vi "打开数据库.vi"(8 "error in (no error)":errorcluster, 11 "sqlerver in":refnum<class "sqlerver.lvclass">) -> (0 "error out":errorcluster, 3 "sqlerver out":refnum<class "sqlerver.lvclass">)   [LabVIEW 2016, in "sqlerver.lvclass"]
uses:
  sqlerver.lvclass
  sqlerver.lvclass/sqlerver.ctl
  <vilib>/addons/database/Connection.llb/DB Tools Open Connec (Path).vi
  <vilib>/addons/database/NI_Database_API.lvlib
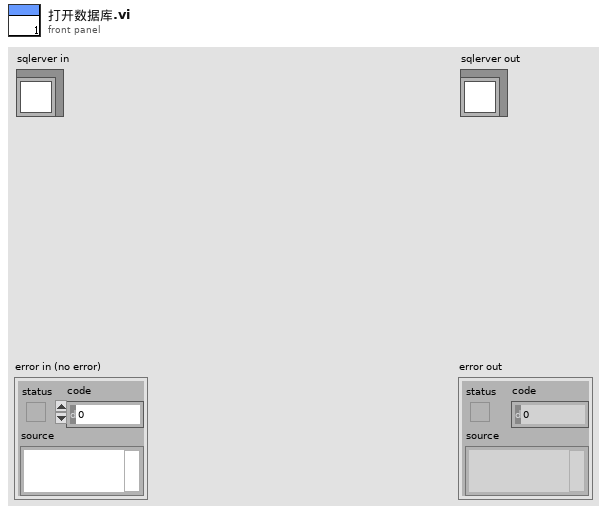
[diagram p1: front panel]
types:
  T1 = typedef "NI_Database_API.lvlib/Conn ObjectReference.ctl" = refnum<k1>
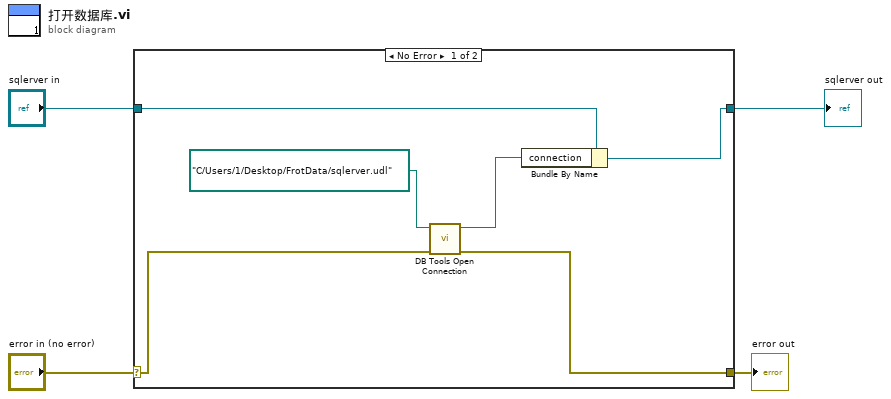
[diagram p0: block diagram]
diagram:
  n1 = case shown="No Error" "error in (no error)" {
    selector: "error in (no error)" -> [w10 w12]
    tunnel: [w9 w12] -> w3
    tunnel: [w5 w11] -> w1
    tunnel: "sqlerver in" -> [w7 w11]
    frame No Error {
      n2 = call-poly <vilib>:"DB Tools Open Connection.vi"("error in (no error)"=w10, "connection information"=path "C:/Users/1/Desktop/FrotData/sqlerver.udl") -> ("error out"=w9:errorcluster, "connection reference"=w6:T1)  [unwired: 6 in]
      n3 = Bundle By Name(cluster=w7, "connection"=w6) -> (w5:refnum<class "sqlerver.lvclass">)
    }
    frame Error {
    }
  }
  "error out" <- w3
  "sqlerver out" <- w1
